vi "VI1.vi"(0 "Cluster":T1 {"Array" format="%.2f"; "Numeric" format="%.2f"}) -> (1 "Numeric":dbl format="%.2f", 2 "String":string, 3 "Array":dbl[](array[numeric]) format="%.2f", 4 "Boolean":bool)   [LabVIEW 2011]
doc: "Unbundles the Data cluster and returns the individual elements"
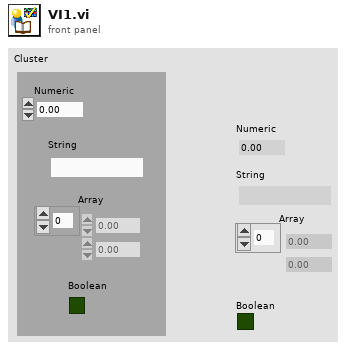
[diagram p1: front panel]
types:
  T1 = cluster{"Numeric":dbl, "String":string, "Array":dbl[], "Boolean":bool}
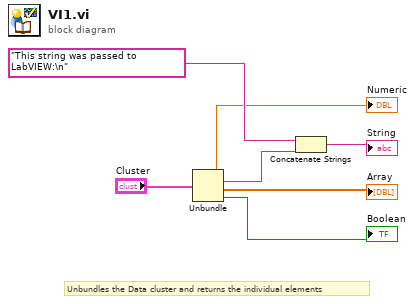
[diagram p0: block diagram]
diagram:
  # "Unbundles the Data cluster and returns the individual elements"
  n1 = Unbundle("Cluster") -> ("Numeric"=→"Numeric":dbl, "String"=w7:string, "Array"=→"Array":dbl[], "Boolean"=→"Boolean":bool)
  n2 = Concatenate Strings("This string was passed to LabVIEW:\n" ("Substring"), w7) -> (→"String":string)
